vi "ComputeKeyFromSeed_BMS.vi"(7 "Session type":T1=enum."Default", 10 "Seed":u8[](array[numeric])=[162, 161, 151, 116] format="%.0x") -> (2 "Key":u8[](array[numeric])=[162, 161, 151, 116] format="%.0x")   [LabVIEW 2020]
uses:
  UDS/Controls/UDS Session Type Cmod.ctl
panel:
  # "BMS\nA2A19774\n\nKEY : A5 D0 40 0A"
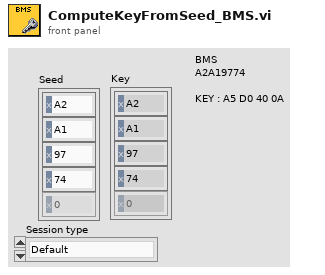
[diagram p1: front panel]
types:
  T1 = typedef "UDS Session Type Cmod.ctl" = enum16{"reserved", "Default", "Programming", "Programming (BMS)", "Extended Diag", "Safety System Diag (BMS)", "Plant (Cmod)", "Garage (Cmod)", "Supplier (Cmod)"}
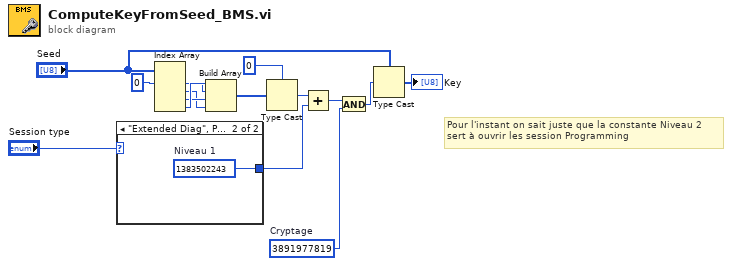
[diagram p0: block diagram]
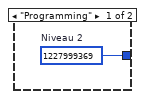
[diagram p2: hidden frame]
diagram:
  w5 = u32 3891977819  # Cryptage
  # "Pour l'instant on sait juste que la constante Niveau 2\nsert à ouvrir les session Programming"
  n1 = case shown="\"Extended Diag\", Par défaut" "Session type" {
    tunnel: [w16 w17] -> w8
    frame "Programming" {
      w16 = u32 1227999369  # Niveau 2
    }
    frame "Extended Diag", Default {
      w17 = u32 1383502243  # Niveau 1
    }
  }
  n2 = Index Array(array="Seed", index #1=0 ("indice")) -> (element #1=w13:u8, element #2=w11:u8, element #3=w12:u8, element #4=w14:u8)  [unwired: 3 in]
  n3 = Build Array(w14, w13, w12, w11) -> (w10:u8[])
  n4 = Type Cast(type=u32 0 ("p_SizeKey"), x=w10) -> (*(type *) &x=w7:u32)
  n5 = Add(x=w7, y=w8) -> (x+y=w6:u32)
  n6 = And(x=w6, y=w5) -> (x .and. y?=w4:u32)
  n7 = Type Cast(type="Seed", x=w4) -> (*(type *) &x=→"Key":u8[])
